vi "LightONsb.vi"() -> ()   [LabVIEW 2015]
uses:
  <vilib>/NXT/Block Support/NXT_InputPort.ctl
  <vilib>/NXT/Block Support/NXT_OutputPort.ctl
  <vilib>/NXT/Dual Mode Library/Sensors/Light_On.vi
  <vilib>/NXT/NXTIO Xnodes/NXTIONodeSubVIs/NXTMoveMotors.vi
  <vilib>/NXT/Dual Mode Library/Waits/Wait_Num(msec).vi
  <vilib>/NXT/NXTIO Xnodes/AddressXNode/NXTIOAddress.xnode
  <vilib>/NXT/Subs/LVHSConnector.ctl
  <vilib>/NXT/NXTIO Xnodes/NXTIOXNode/NXTIO.xnode
  <vilib>/NXT/LegoClasses/BrickReference/BrickReference.lvclass
panel:
  in  "0 speed":i32
  in  "Backward":i32
  in  "Forward":i32
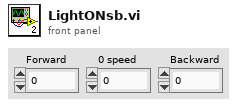
[diagram p1: front panel]
types:
  T1 = typedef "NXT_OutputPort.ctl" = u8
  T2 = typedef "NXT_InputPort.ctl" = u32
  T3 = typedef "LVHSConnector.ctl" = refnum<class "BrickReference.lvclass">
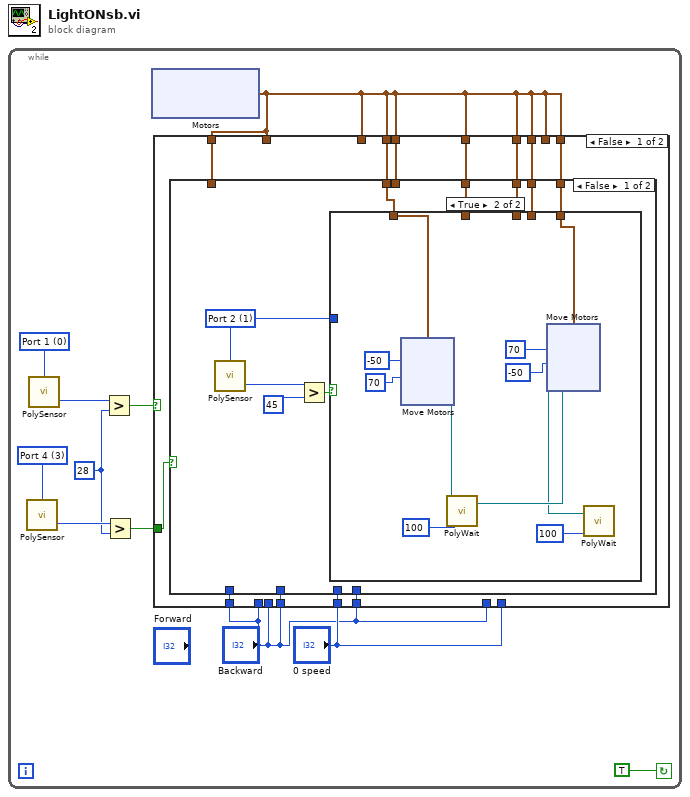
[diagram p0: block diagram]
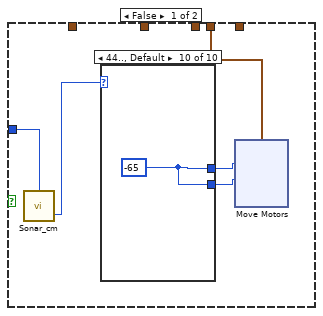
[diagram p2: hidden frame]
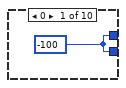
[diagram p3: hidden frame]
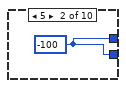
[diagram p4: hidden frame]
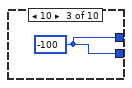
[diagram p5: hidden frame]
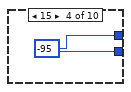
[diagram p6: hidden frame]
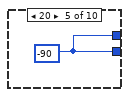
[diagram p7: hidden frame]
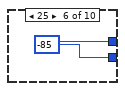
[diagram p8: hidden frame]
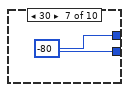
[diagram p9: hidden frame]
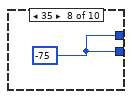
[diagram p10: hidden frame]
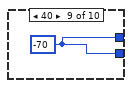
[diagram p11: hidden frame]
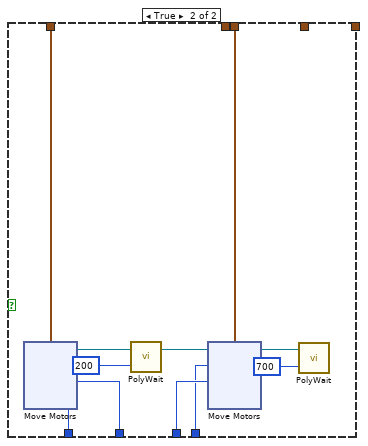
[diagram p12: hidden frame]
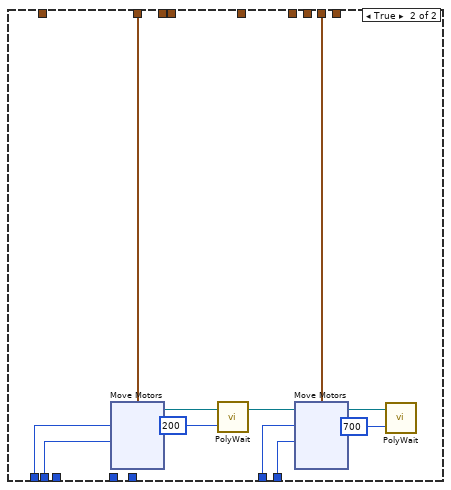
[diagram p13: hidden frame]
diagram:
  n1 = while {
    stop <- TRUE continue-if-true
    w7 = 28
    w10 = T2 3 items=["Port 1", "Port 2", "Port 3", "Port 4"] ("Port (Port 3)")
    w11 = T2 0 items=["Port 1", "Port 2", "Port 3", "Port 4"] ("Port (Port 3)")
    n2 = call-poly <vilib>:"PolySensor.vi"("Port (Port 3)"=w10) -> ("Scaled Value"=w9:i16)  [unwired: 2 in, 1 out]
    n3 = call-poly <vilib>:"PolySensor.vi"("Port (Port 3)"=w11) -> ("Scaled Value"=w8:i16)  [unwired: 2 in, 1 out]
    n4 = Greater?(x=w8, y=w7) -> (0:w5:bool)
    n5 = Greater?(x=w9, y=w7) -> (0:w4:bool)
    n6 = xnode "Motors"() -> ("Motor"=w1:cluster{"Port":T1, "Port":T1})
    n7 = case shown="False" w5 {
      tunnel: "Backward" -> [_ w119]
      tunnel: "Backward" -> [_ w112]
      tunnel: "0 speed" -> [_ w111]
      tunnel: "Backward" -> [_ w117]
      tunnel: w1 -> [_ w114]
      tunnel: w1 -> [_ w113]
      tunnel: w1 -> [_ _]
      tunnel: w4 -> [w24 _]
      tunnel: w1 -> [w23 _]
      tunnel: w1 -> [w22 _]
      tunnel: "0 speed" -> [w21 _]
      tunnel: "Backward" -> [w20 _]
      tunnel: "Backward" -> [w19 _]
      tunnel: "Backward" -> [w18 _]
      tunnel: w1 -> [w17 _]
      tunnel: w1 -> [w16 _]
      tunnel: w1 -> [w15 _]
      tunnel: w1 -> [w14 _]
      tunnel: w1 -> [w13 _]
      frame False {
        n8 = case shown="False" w24 {
          tunnel: w23 -> [_ w94]
          tunnel: w22 -> [_ w93]
          tunnel: w21 -> [_ w87]
          tunnel: w20 -> [_ w86]
          tunnel: w19 -> [_ w85]
          tunnel: w18 -> [_ w84]
          tunnel: w17 -> [w30 _]
          tunnel: w16 -> [w29 _]
          tunnel: w15 -> [w28 _]
          tunnel: w14 -> [w27 _]
          tunnel: w13 -> [w25 _]
          frame False {
            w26 = T2 1 items=["Port 1", "Port 2", "Port 3", "Port 4"] ("Port (Port 4)")
            n9 = call-poly <vilib>:"PolySensor.vi"("Port (Port 4)"=w26) -> ("Distance (cm)"=w32:i16)  [unwired: 2 in, 1 out]
            n10 = Greater?(x=w32, y=45) -> (0:w31:bool)
            n11 = case shown="True" w31 {
              tunnel: w30 -> [_ w67]
              tunnel: w29 -> [_ w64]
              tunnel: w28 -> [_ _]
              tunnel: w27 -> [_ _]
              tunnel: w26 -> [w35 _]
              tunnel: w25 -> [w38 _]
              frame False {
                n12 = call <vilib>:"Sonar_cm.vi"("Port (Port 4)"=w35) -> ("Distance (cm)"=w34:i16)  [unwired: 2 in, 1 out]
                n13 = case shown="44.., Default" w34 {
                  tunnel: [w47 w48 w49 w50 w51 w52 w53 w54 w55 w56] -> w37
                  tunnel: [w47 w48 w49 w50 w51 w52 w53 w54 w55 w56] -> w36
                  frame 0 {
                    w47 = -100
                  }
                  frame 5 {
                    w48 = -100
                  }
                  frame 10 {
                    w49 = -100
                  }
                  frame 15 {
                    w50 = -95
                  }
                  frame 20 {
                    w51 = -90
                  }
                  frame 25 {
                    w52 = -85
                  }
                  frame 30 {
                    w53 = -80
                  }
                  frame 35 {
                    w54 = -75
                  }
                  frame 40 {
                    w55 = -70
                  }
                  frame 44.., Default {
                    w56 = -65
                  }
                }
                n14 = xnode "Move Motors"("Power/Speed 2"=w36, "Power/Speed 1"=w37, "Motors"=w38) -> ()  [unwired: 1 in, 1 out]
              }
              frame True {
                n15 = xnode "Move Motors"("Power/Speed 2"=70, "Power/Speed 1"=-50, "Motors"=w67) -> ("NXT/EV3"=w66:T3)  [unwired: 1 in]
                n16 = call-poly <vilib>:"PolyWait.vi"("Time (100 msec)"=100, "NXT/EV3"=w66) -> ("NXT/EV3"=w65:T3)  [unwired: 2 in]
                n17 = xnode "Move Motors"("Power/Speed 2"=-50, "Power/Speed 1"=70, "Motors"=w64, "NXT/EV3"=w65) -> ("NXT/EV3"=w62:T3)
                n18 = call-poly <vilib>:"PolyWait.vi"("Time (100 msec)"=100, "NXT/EV3"=w62) -> ()  [unwired: 2 in, 1 out]
              }
            }
          }
          frame True {
            n19 = xnode "Move Motors"("Power/Speed 2"=w84, "Power/Speed 1"=w85, "Motors"=w94) -> ("NXT/EV3"=w92:T3)  [unwired: 1 in]
            n20 = call-poly <vilib>:"PolyWait.vi"("Time (100 msec)"=200, "NXT/EV3"=w92) -> ("NXT/EV3"=w91:T3)  [unwired: 2 in]
            n21 = xnode "Move Motors"("Power/Speed 2"=w87, "Power/Speed 1"=w86, "Motors"=w93, "NXT/EV3"=w91) -> ("NXT/EV3"=w90:T3)
            n22 = call-poly <vilib>:"PolyWait.vi"("Time (100 msec)"=700, "NXT/EV3"=w90) -> ()  [unwired: 2 in, 1 out]
          }
        }
      }
      frame True {
        n23 = xnode "Move Motors"("Power/Speed 2"=w112, "Power/Speed 1"=w119, "Motors"=w114) -> ("NXT/EV3"=w121:T3)  [unwired: 1 in]
        n24 = call-poly <vilib>:"PolyWait.vi"("Time (100 msec)"=200, "NXT/EV3"=w121) -> ("NXT/EV3"=w120:T3)  [unwired: 2 in]
        n25 = xnode "Move Motors"("Power/Speed 2"=w111, "Power/Speed 1"=w117, "Motors"=w113, "NXT/EV3"=w120) -> ("NXT/EV3"=w116:T3)
        n26 = call-poly <vilib>:"PolyWait.vi"("Time (100 msec)"=700, "NXT/EV3"=w116) -> ()  [unwired: 2 in, 1 out]
      }
    }
  }
